vi "1DArrayToNode(viaString).vi"(0 "Tree DVR in":refnum<data-value>, 1 "DBL Array":dbl[](array[numeric]), 3 "error in (no error)":errorcluster, 4 "NodePath":string) -> (5 "Tree DVR out":refnum<data-value>, 6 "TreeNode DVR out":refnum<data-value>, 7 "error out":errorcluster)   [LabVIEW 2013]
uses:
  <vilib>/MDSplus/Classes/Tree_Class/Tree.lvclass
  <vilib>/MDSplus/Classes/Data_Class/TreeNode_Class/TreeNode.lvclass
  <vilib>/MDSplus/Library/MDSplus.lvlib
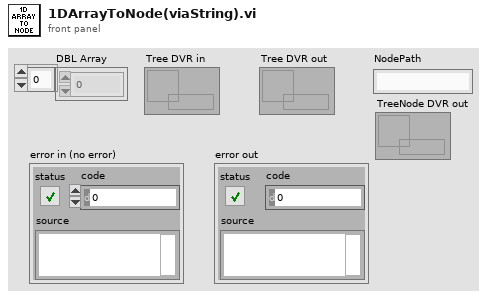
[diagram p1: front panel]
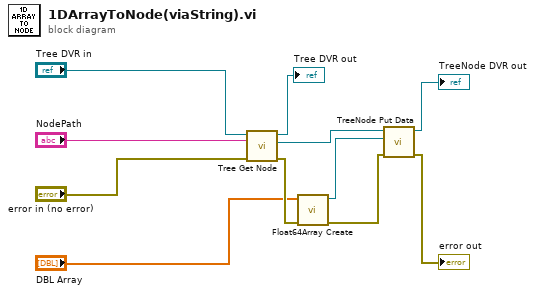
[diagram p0: block diagram]
diagram:
  n1 = call <vilib>:"Tree Get Node.vi"("error in (no error)"="error in (no error)", "Path"="NodePath", "Tree DVR in"="Tree DVR in") -> ("error out"=w7:errorcluster, "Node out"=w6:refnum<data-value>, "Tree DVR out"=→"Tree DVR out":refnum<data-value>)  [unwired: 6 in]
  n2 = call <vilib>:"Float64Array Create.vi"("error in (no error)"=w7, "DBL array in"="DBL Array") -> ("error out"=w4:errorcluster, "Float64Array DVR out"=w5:refnum<data-value>)  [unwired: 8 in]
  n3 = call <vilib>:"TreeNode Put Data.vi"("error in (no error)"=w4, "Data"=w5, "TreeNode DVR in"=w6) -> ("error out"=→"error out":errorcluster, "TreeNode DVR out"=→"TreeNode DVR out":refnum<data-value>)  [unwired: 7 in]
